vi "Add Records.vi"(7 "Bulk Insert?":bool, 8 "Error In (no error)":errorcluster, 10 "Expenses Tracker Records In":refnum<class "Expenses Tracker Record.lvclass">[](array[class]), 11 "Database Interactions In":refnum<class "Database Interactions.lvclass">) -> (0 "Error Out":errorcluster, 2 "Expenses Tracker Records Out":refnum<class "Expenses Tracker Record.lvclass">[](array[class]), 3 "Database Interactions Out":refnum<class "Database Interactions.lvclass">)   [LabVIEW 2023, in "Database Interactions.lvclass"]
uses:
  Database Interactions.lvclass
  Expenses Tracker Record/Expenses Tracker Record.lvclass
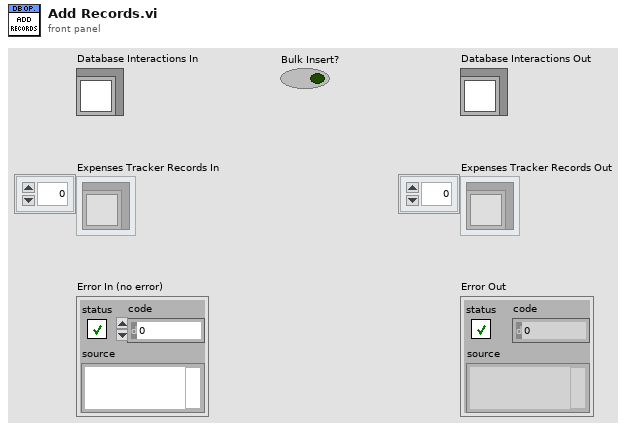
[diagram p1: front panel]
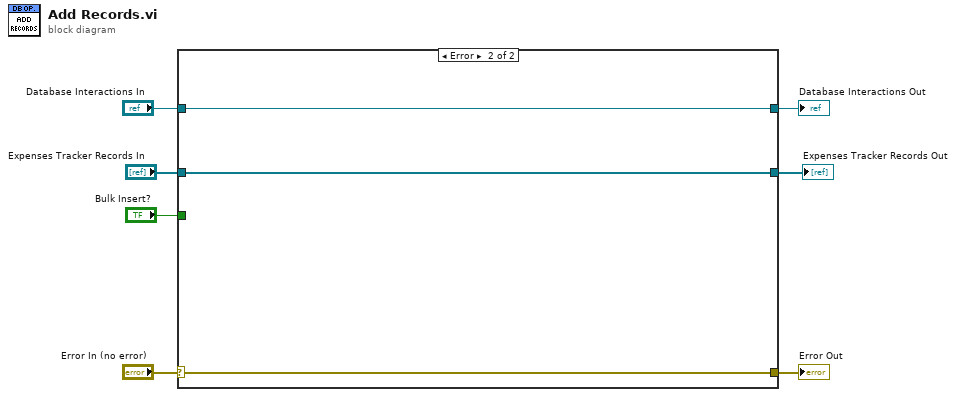
[diagram p0: block diagram]
diagram:
  n1 = case shown="Error" "Error In (no error)" {
    selector: "Error In (no error)" -> [w9 w13]
    tunnel: [w9 w13] -> w6
    tunnel: [w10 w12] -> w4
    tunnel: "Database Interactions In" -> [w10 w12]
    tunnel: "Expenses Tracker Records In" -> [w8 w11]
    tunnel: [w8 w11] -> w2
    tunnel: "Bulk Insert?" -> [_ _]
    frame No Error {
      # "Wire the error cluster across even in the \"No Error\"\ncase so that warnings get propagated."
    }
    frame Error {
    }
  }
  "Error Out" <- w6
  "Database Interactions Out" <- w4
  "Expenses Tracker Records Out" <- w2
